vi "debugKickValue.vi"(8 "error in (no error)":errorcluster, 10 "RoboRefArray in":refnum<class "Robot.lvclass">[](array[class]), 11 "Game in":refnum<class "Game.lvclass">) -> (0 "error out":errorcluster, 2 "RoboRefArray out":refnum<class "Robot.lvclass">[](array[class]), 3 "Game out":refnum<class "Game.lvclass">)   [LabVIEW 2023, in "Game.lvclass"]
uses:
  Game.lvclass
  Robot_class/Robot.lvclass
  Game.lvclass/Game.ctl
  Parameters_class/Parameters.lvclass/Parameters.ctl
  Robot_class/Robot.lvclass/Robot.ctl
  Robot_class/Write v_tang.vi
  Robot_class/Write v_norm.vi
  Robot_class/Write v_ang.vi
  Robot_class/Write kick_x.vi
  Read Parameters.lvclass.vi
  Parameters_class/Read Debug.vi
  Parameters_class/Parameters.lvclass
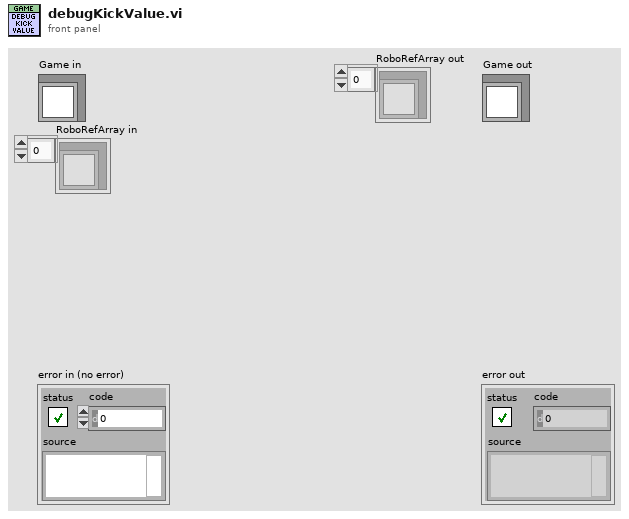
[diagram p1: front panel]
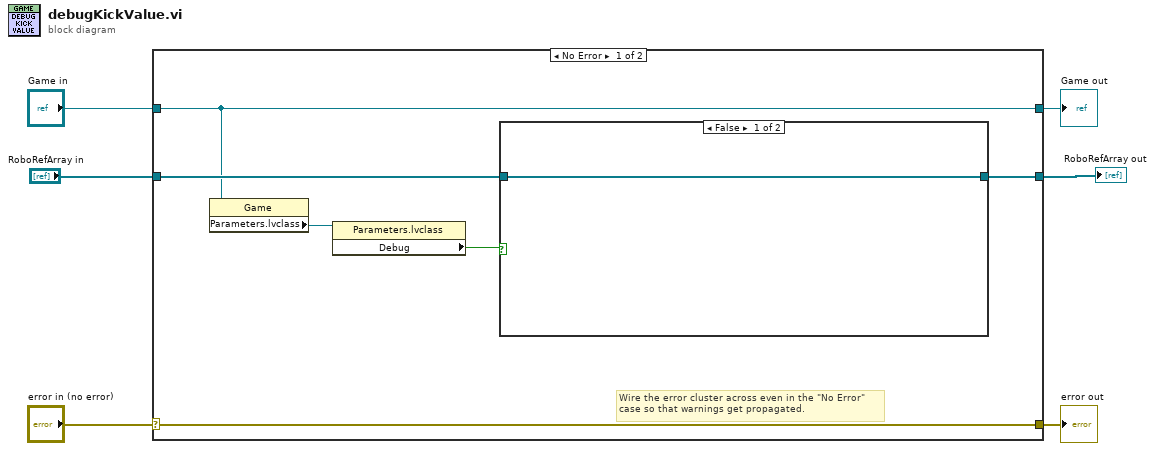
[diagram p0: block diagram]
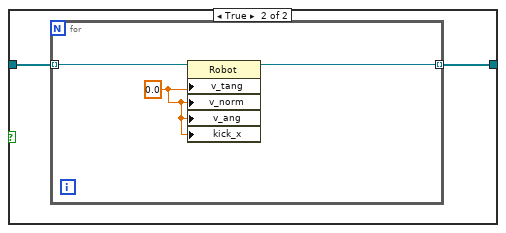
[diagram p2: hidden frame]
diagram:
  n1 = case shown="No Error" "error in (no error)" {
    selector: "error in (no error)" -> [w12 w20]
    tunnel: [w12 w20] -> w5
    tunnel: [w9 w19] -> w3
    tunnel: "Game in" -> [w9 w19]
    tunnel: "RoboRefArray in" -> [w11 _]
    tunnel: [w10 _] -> w1
    frame No Error {
      # "Wire the error cluster across even in the \"No Error\"\ncase so that warnings get propagated."
      n2 = property class="Game"(reference=w9) -> ("Parameters.lvclass"=w8:refnum<class "Parameters.lvclass">)  [unwired: 1 in, 2 out]
      n3 = property class="Parameters.lvclass"(reference=w8) -> ("Debug"=w7:bool)  [unwired: 1 in, 2 out]
      n4 = case shown="False" w7 {
        tunnel: w11 -> [w13 w15]
        tunnel: [w13 w14] -> w10
        frame False {
        }
        frame True {
          n5 = for {
            tunnel: w15 -> [w18] mode=indexing
            tunnel: [w17] -> w14 mode=indexing
            w16 = 0.0
            n6 = property class="Robot"(reference=w18, "v_tang"=w16, "v_norm"=w16, "v_ang"=w16, "kick_x"=w16) -> (reference out=w17:refnum<class "Robot.lvclass">)  [unwired: 1 in, 1 out]
          }
        }
      }
    }
    frame Error {
    }
  }
  "error out" <- w5
  "Game out" <- w3
  "RoboRefArray out" <- w1
